vi "Dashboard Main.vi"() -> ()   [LabVIEW 2017]
uses:
  <vilib>/event_ctls.llb/eventvkey.ctl
  <vilib>/Rock Robotics/WPI/Dashboard/WPI_DashboardLogging Global.vi
  <vilib>/Utility/miscctls.llb/LVRowAndColumnTypeDef.ctl
  <vilib>/Rock Robotics/Network Tables/NT Read Boolean.vi
  <vilib>/Rock Robotics/Network Tables/NT Read Numeric Array.vi
panel:
  in  "Camera Settings Right":T1={"Frame Rate"=30, "Compression"=30, "Size"=1, "DB Camera Config"=FALSE} {"Frame Rate" scale=1.0..30.0; "Compression" scale=100.0..-1.0; "Size" items=["640x480", "320x240", "160x120"]}
  in  "Camera Name Right":string(combo)="No Camera Selection"
  out "Camera Info":cluster{"Mbps LED":bool, "Mbps":dbl, "fps":dbl} {"fps" format="%#.1g"; "Mbps" format="%#.1g"}
  in  "Camera Settings":T1={"Frame Rate"=30, "Compression"=30, "Size"=1, "DB Camera Config"=FALSE} {"Frame Rate" scale=1.0..30.0; "Compression" scale=100.0..-1.0; "Size" items=["640x480", "320x240", "160x120"]}
  in  "TCP":refnum<k5>
  in  "Rec Mode":enum32{"Stop", "Record", "Playback"}(radio)
  out "Robot IP":string
  out "Image Message":string="Timeout in Camera Communications"
  in  "Dashboard Tab":T2(tab)
  in  "Select Auto":string(combo)="Select Autonomous ..."
  out "NT Connection":bool
  out "MotorChart R":cluster{"Numeric":dbl, "Numeric":dbl}(graph)
  out "MotorChart L":cluster{"Numeric":dbl, "Numeric":dbl}(graph)
  out "MotorSliders R":cluster{"MotorSlide1":dbl, "MotorSlide2":dbl} {"MotorSlide2" scale=-1.0..1.0 scale format="%#_2e"; "MotorSlide1" scale=-1.0..1.0 scale format="%#_2e"}
  out "MotorSliders L":cluster{"MotorSlide1":dbl, "MotorSlide2":dbl} {"MotorSlide2" scale=-1.0..1.0 scale format="%#_2e"; "MotorSlide1" scale=-1.0..1.0 scale format="%#_2e"}
  out "JS1 Z":dbl(slide) scale=-1.0..1.0 scale format="%#_2e"
  out "JS1 Graph":cluster{"X":dbl, "Y":dbl}[](graph)
  out "JS1 Buttons":T3
  out "JS2 Z":dbl(slide) scale=-1.0..1.0 scale format="%#_2e"
  out "JS2 Graph":cluster{"X":dbl, "Y":dbl}[](graph)
  out "JS2 Buttons":T3
  out "Mode":T4(ring)=enum."Auto Disabled"
  out "Camera Image Right":T5(plugin-control)
  in  "DB/String 9":string
  in  "DB/String 8":string
  in  "DB/String 7":string
  in  "DB/String 6":string
  in  "DB/String 5":string
  in  "DB/String 4":string
  in  "DB/String 3":string
  in  "DB/String 2":string
  in  "DB/String 1":string
  in  "DB/String 0":string
  in  "DB/Slider 0":dbl(slide) scale=0.0..5.0
  in  "DB/Slider 1":dbl(slide) scale=0.0..5.0
  in  "DB/Slider 2":dbl(slide) scale=0.0..5.0
  in  "DB/Slider 3":dbl(slide) scale=0.0..5.0
  out "DB/LED 3":bool
  out "DB/LED 2":bool
  out "DB/LED 1":bool
  out "DB/LED 0":bool
  in  "DB/Button 3":bool
  in  "DB/Button 2":bool
  in  "DB/Button 1":bool
  in  "DB/Button 0":bool caption="New Name"
  in  "Test Slider":dbl(slide) scale=0.0..100.0 scale format="%#_3g"
  in  "On/Off":bool caption="Solenoid"
  in  "Test Name":u16(ring) items=["Select the test to run..."]
  in  "Test Tree":string(tree)
  in  "Motor":cluster{"Value":dbl, "Enable":bool} {"Value" scale=-1.0..1.0 scale format="%#_3g"}
  out "Progress":T6 {"Test Progress" scale=0.0..100.0}
  in  "Rev/Fwd":cluster{"Forward":bool, "Reverse":bool}
  in  "Test Ring":u16(ring) items=["Monochrome", "Color"]
  out "Cmd Status":string
  in  "Execute Command":bool
  in  "Command Params":string[][](table)
  in  "Command Selection":i32(listbox)
  in  "CheckList":i32(listbox)
  out "Tree":string(tree)
  out "Camera Image":T5(plugin-control)
  out "Background":bool
  in  "Camera Name":string(combo)="No Camera Selection"
  # "HW"
  # "HW"
  # "Drive Motors"
  # "Joysticks"
  # "Front"
  # "Right"
  # "Left"
  # "Back"
  # "This tab is a great place for autonomous settings and robot-specific values.\nPlace controls and indicators inside this tab and match name to\nDashboard Variables on robot. You can also delete this comment."
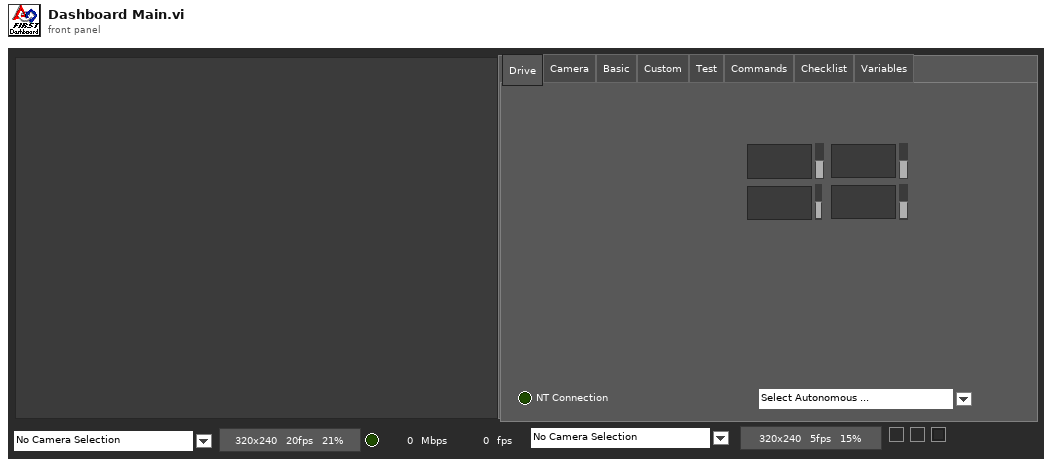
[diagram p1: front panel]
types:
  T1 = cluster{"Frame Rate":i32, "Compression":i32, "Size":u16, "DB Camera Config":bool}
  T2 = enum32{"Drive", "Camera", "Basic", "Custom", "Test", "Commands", "Checklist", "Variables"}
  T3 = cluster{bool, bool, bool, bool, bool, bool, bool, bool, bool, bool, bool, bool}
  T4 = enum8{"Tele-Op Disabled", "Tele-Op Enabled", "Auto Disabled", "Auto Enabled", "Test Disabled", "Test Enabled", "Disconnected", "No Code", "E-Stop"}
  T5 = typedef "IMAQ Image.ctl" = refnum<image>
  T6 = cluster{"Test Progress":u8, "Test Progress Text":string}
  T7 = cluster{"Save Path":path, "Interval (s)":dbl, "Keep":i32}
  T8 = typedef "Image Type" = u32
  T9 = cluster{"IDs":cluster{"RPC field ID":u16, "Unique ID":u16}, "String":string}
  T10 = cluster{"Error Strings":string, "Disable Counts":cluster{u16, u16}, "Rail Faults":cluster{u16, u16, u16}, "Robot IP":string, "DB Mode":u8, "Event Info":cluster{"Name":string, "Type":u8, "Number":u16, "Replay":u8}}
  T11 = cluster{"Storage":cluster{"Disk Free":u64, "RAM Block":u32, "RAM free":u32}, "CPU Utilization":cluster{"CPU % ISR":sgl, "CPU % Time Crit":sgl, "CPU % Timed Str":sgl, "CPU % High":sgl, "CPU % Above":sgl, "CPU % Normal":sgl, "CPU % Low":sgl}, "CAN":cluster{"% Bus Utilization":sgl, "Bus Off Cnt":u32, "TX_FIFO Full Cnt":u32, "Receive Error Cnt":u8, "Transmit Error Cnt":u8}, "HID":cluster{"HID Outputs":u32, "Rumble Low":u16, "Rumble High":u16}[]}
  T12 = cluster{"Status bits":cluster{"Test Mode":bool, "Autonomous":bool, "Enabled":bool, "Code Start":bool, "Brownout":bool, "Reserved 2":bool, "Reserved 3":bool, "E-Stop":bool}, "Code Trace":cluster{"Disabled":bool, "TeleOp":bool, "Auto":bool, "Test":bool}, "Controller Type":enum16{"unknown", "cRIO", "roboRio"}, "Code?":enum16{"unknown", "noCode", "code"}, "Battery V":dbl}
  T13 = cluster{"Control Bits":cluster{"TestMode":bool, "Autonomous":bool, "Enabled":bool, "FMS Present":bool, bool, bool, bool, "E-Stop":bool}, "Team Station ":u8, "Countdown":sgl, "Joystick Values":cluster{"Axes":dbl[], "Buttons":bool[], "POVs":i16[]}[]}
  T14 = cluster{"Axes":dbl[], "Buttons":bool[], "POVs":i16[]}[]
  T15 = cluster{"Axes":dbl[], "Buttons":bool[], "POVs":i16[]}
  T16 = cluster{"Buttons[0]":bool, "Buttons[1]":bool, "Buttons[2]":bool, "Buttons[3]":bool, "Buttons[4]":bool, "Buttons[5]":bool, "Buttons[6]":bool, "Buttons[7]":bool, "Buttons[8]":bool, "Buttons[9]":bool, "Buttons[10]":bool, "Buttons[11]":bool}
  T17 = cluster{"Camera Image":refnum<vi>, "Dashboard Tab":refnum<vi>, "Background":refnum<vi>, "Rec Mode":refnum<vi>, "Test Slider":refnum<vi>, "On/Off ":refnum<vi>, "Test Ring":refnum<vi>, "Rev/Fwd":refnum<vi>, "Test Name":refnum<vi>, "Motor":refnum<vi>, "Progress":refnum<vi>, "CheckList":refnum<vi>, "Tree":refnum<vi>, "Test Tree":refnum<vi>, "Command Params":refnum<vi>, "Command Selection":refnum<vi>, "Execute Command":refnum<vi>, "Cmd Status":refnum<vi>, "Camera Settings":refnum<vi>, "Camera Name":refnum<vi>, "Camera Info":refnum<vi>, "Camera Settings Right":refnum<vi>, "Camera Name Right":refnum<vi>, "Camera Image Right":refnum<vi>}
  T18 = cluster{"Camera Name":string, string, "Saved DB Images Info":cluster{"Save Path":path, "Interval (s)":dbl, "Keep":i32}}
  T19 = cluster{"Camera Name Right":string, string, "Saved DB Images Info":cluster{"Save Path":path, "Interval (s)":dbl, "Keep":i32}}
  T20 = cluster{"Operation":enum16{"Update", "Clear"}, "Color Box":u32}[]
  T21 = typedef "eventvkey.ctl" = enum16{"ASCII", "Enter", "Return", "Shift", "Ctrl", "Alt", "Cmd", "Opt", "Caps", "NumLock", "Clear", "Break", "Up", "Down", "Left", "Right", "Insert", "Delete", "Home", "End", "PageUp", "PageDown", "Escape", "Help", "Pause", "ScrollLock", "F1", "F2", "F3", "F4", "F5", "F6", "F7", "F8", "F9", "F10", "F11", "F12", "F13", "F14", "F15", "F16", "F17", "F18", "F19", "F20", "F21", "F22", "F23", "F24", "Play", "VolumeUp", "VolumeDown", "Mute", "Two Byte Char"}
  T22 = cluster{"Image Size":bool, "Image Type":bool, "Pixel Value":bool, "ROI Information":bool, "Zoom Factor":bool}
  T23 = cluster{"Operation":enum16{"Update", "Clear"}, "Color Box":u32}
  T24 = typedef "LVRowAndColumnTypeDef.ctl" = cluster{"Row":i32, "Column":i32}
  T25 = cluster{"Shift":bool, "Ctrl":bool, "Alt":bool, "Cmd":bool, "Opt":bool}
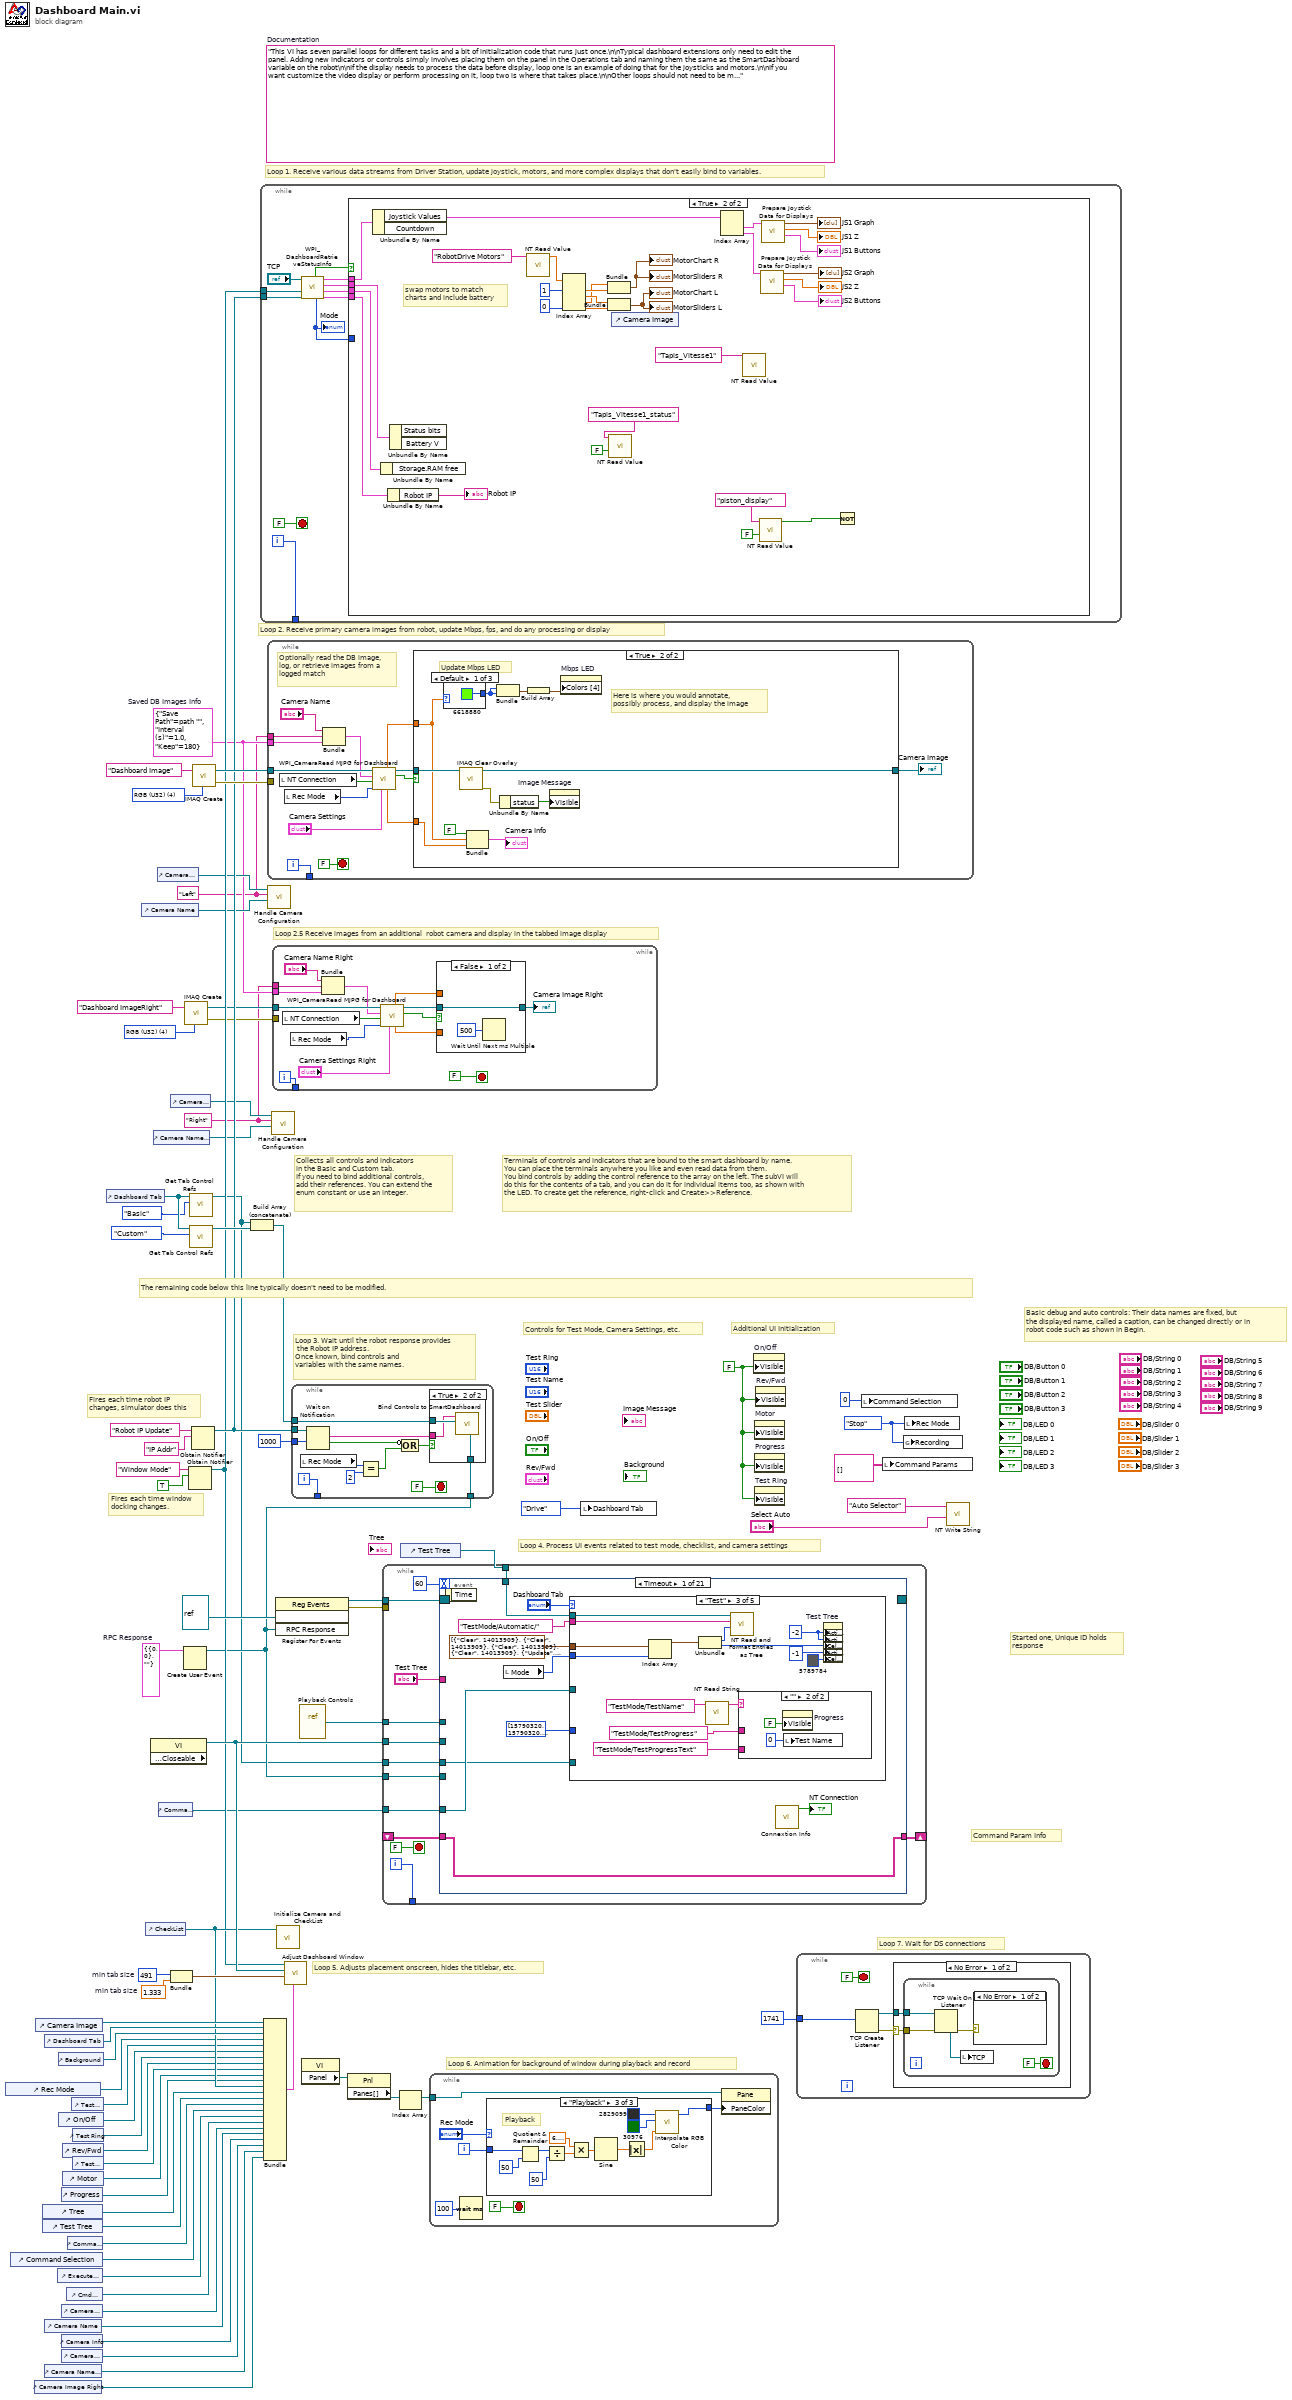
[diagram p0: block diagram]
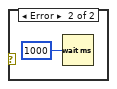
[diagram p3: hidden frame]
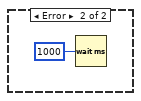
[diagram p4: hidden frame]
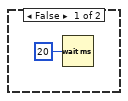
[diagram p5: hidden frame]
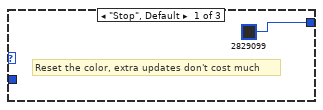
[diagram p6: hidden frame]
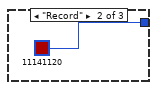
[diagram p7: hidden frame]
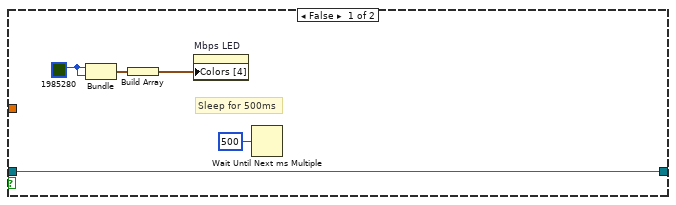
[diagram p9: hidden frame]
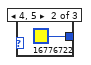
[diagram p10: hidden frame]
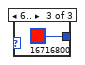
[diagram p11: hidden frame]
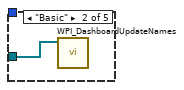
[diagram p13: hidden frame]
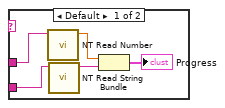
[diagram p14: hidden frame]
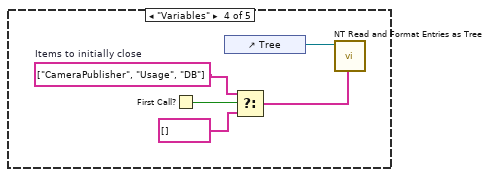
[diagram p15: hidden frame]
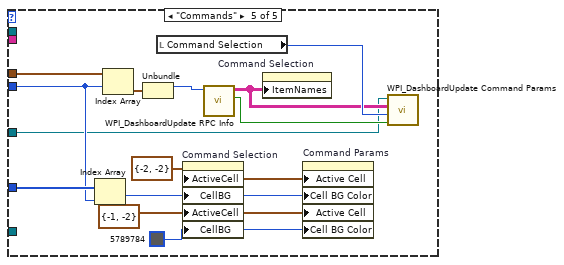
[diagram p16: hidden frame]
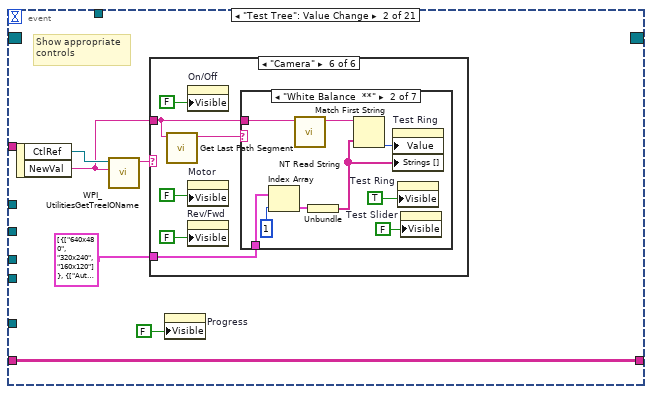
[diagram p17: hidden frame]
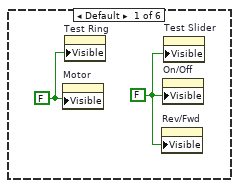
[diagram p18: hidden frame]
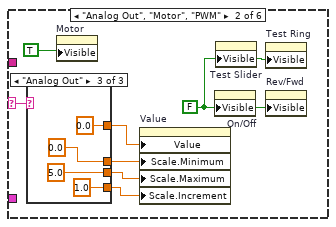
[diagram p19: hidden frame]
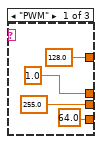
[diagram p20: hidden frame]
diagram:
  w3 = T7 {"Save Path"=path "", "Interval (s)"=1.0, "Keep"=180}  # Saved DB Images Info
  w2 = "Right"
  w1 = "Left"
  w13 = T8 4 items=["Grayscale (U8)", "Grayscale (I16)", "Grayscale (SGL)", "Complex (CSG)", "RGB (U32)", "HSL (U32)", "RGB (U64)"] ("Image Type")
  w29 = T9 {"IDs"={"RPC field ID"=0, "Unique ID"=0}, "String"=""}  # RPC Response
  w52 = 491  # min tab size
  w51 = 1.333  # min tab size
  w59 = enum32{"Stop", "Record", "Playback"}."Stop" ("Rec Mode")
  w36 = FALSE ("Visible")
  (unwired) "This VI has seven parallel loops for different tasks and a bit of initialization code that runs just once.\n\nTypical dashboard extensions only need to edit the panel. Adding new indicators or controls simply involves placing them on the panel in the Operations tab and naming them the same as the SmartDashboard variable on the robot\n\nIf the display needs to process the data before display, loop one is an example of doing that for the joysticks and motors.\n\nIf you want customize the video display or perform processing on it, loop two is where that takes place.\n\nOther loops should not need to be modified. They are pretty standard, and document the task they perform."  # Documentation
  w76 = T8 4 items=["Grayscale (U8)", "Grayscale (I16)", "Grayscale (SGL)", "Complex (CSG)", "RGB (U32)", "HSL (U32)", "RGB (U64)"] ("Image Type")
  # "Loop 2.5 Receive images from an additional  robot camera and display in the tabbed image display"
  # "Command Param Info"
  # "Started one, Unique ID holds\nresponse"
  # "Loop 7. Wait for DS connections"
  # "Basic debug and auto controls: Their data names are fixed, but\nthe displayed name, called a caption, can be changed directly or in\nrobot code such as shown in Begin."
  # "Controls for Test Mode, Camera Settings, etc."
  # "Additional UI Initialization"
  # "Loop 6. Animation for background of window during playback and record"
  # "Fires each time robot IP\nchanges, simulator does this"
  # "Fires each time window\ndocking changes."
  # "Collects all controls and indicators\nin the Basic and Custom tab.\nIf you need to bind additional controls,\nadd their references. You can extend the\nenum constant or use an integer."
  # "The remaining code below this line typically doesn't need to be modified."
  # "Loop 4. Process UI events related to test mode, checklist, and camera settings"
  # "Terminals of controls and indicators that are bound to the smart dashboard by name.\nYou can place the terminals anywhere you like and even read data from them.\nYou bind controls by adding the control reference to the array on the left. The subVI will\ndo this for the contents of a tab, and you can do it for individual items too, as shown with\nthe LED. To create get the reference, right-click and Create>>Reference."
  # "Loop 3. Wait until the robot response provides\n the Robot IP address.\nOnce known, bind controls and\nvariables with the same names."
  # "Loop 5. Adjusts placement onscreen, hides the titlebar, etc."
  # "Loop 1. Receive various data streams from Driver Station, update joystick, motors, and more complex displays that don't easily bind to variables."
  # "Loop 2. Receive primary camera images from robot, update Mbps, fps, and do any processing or display"
  n1 = control-ref of="Rec Mode"() -> (w42:refnum<vi>)
  n2 = control-ref of="Command Selection"() -> (w28:refnum<vi>)
  n3 = control-ref of="Camera Image Right"() -> (w6:refnum<vi>)
  n4 = control-ref of="Camera Image"() -> (w54:refnum<vi>)
  n5 = control-ref of="Tree"() -> (w46:refnum<vi>)
  n6 = control-ref of="Test Tree"() -> (w45:refnum<vi>)
  n7 = control-ref of="Dashboard Tab"() -> (w53:refnum<vi>)
  n8 = control-ref of="Camera Name"() -> (w19:refnum<vi>)
  n9 = control-ref of="Camera Name Right"() -> (w7:refnum<vi>)
  n10 = control-ref of="Execute Command"() -> (w30:refnum<vi>)
  n11 = control-ref of="Background"() -> (w49:refnum<vi>)
  n12 = control-ref of="On/Off"() -> (w40:refnum<vi>)
  n13 = control-ref of="Progress"() -> (w37:refnum<vi>)
  n14 = control-ref of="Camera Settings"() -> (w20:refnum<vi>)
  n15 = control-ref of="Camera Info"() -> (w18:refnum<vi>)
  n16 = control-ref of="Camera Settings Right"() -> (w8:refnum<vi>)
  n17 = control-ref of="Rev/Fwd"() -> (w38:refnum<vi>)
  n18 = control-ref of="Motor"() -> (w43:refnum<vi>)
  n19 = control-ref of="Cmd Status"() -> (w24:refnum<vi>)
  n20 = control-ref of="Command Params"() -> (w31:refnum<vi>)
  n21 = control-ref of="Test Slider"() -> (w41:refnum<vi>)
  n22 = control-ref of="Test Ring"() -> (w39:refnum<vi>)
  n23 = control-ref of="Test Name"() -> (w44:refnum<vi>)
  n24 = control-ref of="Dashboard Tab"() -> (w57:refnum<vi>)
  n25 = control-ref of="Camera Name"() -> (w21:refnum<vi>)
  n26 = control-ref of="CheckList"() -> (w47:refnum<vi>)
  n27 = property class="VI" props=["Front Panel.Closeable"]() -> (reference out=w58:refnum<vi>)  [unwired: 2 in, 2 out]
  n28 = control-ref of="Camera Name Right"() -> (w9:refnum<vi>)
  n29 = control-ref of="Camera Settings"() -> (w22:refnum<vi>)
  n30 = control-ref of="Command Params"() -> (w23:refnum<vi>)
  n31 = control-ref of="Camera Settings Right"() -> (w10:refnum<vi>)
  n32 = Bundle("min tab size"=w52, "min tab size"=w51) -> (w50:cluster{"min tab size":i32, "min tab size":dbl})  [unwired: 1 in]
  n33 = Create User Event(user event datatype=w29) -> (user event=w25:refnum<user-event>)  [unwired: 1 in, 1 out]
  n34 = call "IMAQ Create"("Image Name"="Dashboard ImageRight", "Image Type"=w13) -> ("New Image"=w12:T5, "error out"=w11:errorcluster)  [unwired: 2 in, 1 out]
  n35 = Obtain Notifier(name (unnamed)="Window Mode", notification data type=TRUE) -> (notifier out=w34:refnum<notifier>)  [unwired: 2 in, 2 out]
  n36 = call <vilib>:"Get Tab Control Refs.vi"("Page Index"=T2."Basic" ("Dashboard Tab"), "TabControl in"=w57) -> ("ControlsOnPage"=w17:refnum<vi>[])  [unwired: 9 in]
  n37 = call <vilib>:"Get Tab Control Refs.vi"("Page Index"=T2."Custom" ("Dashboard Tab"), "TabControl in"=w57) -> ("ControlsOnPage"=w56:refnum<vi>[])  [unwired: 9 in]
  n38 = Obtain Notifier(name (unnamed)="Robot IP Update", notification data type="IP Addr" ("name (unnamed)")) -> (notifier out=w35:refnum<notifier>)  [unwired: 2 in, 2 out]
  n39 = call "IMAQ Create"("Image Name"="Dashboard Image", "Image Type"=w76) -> ("New Image"=w74:T5, "error out"=w73:errorcluster)  [unwired: 2 in, 1 out]
  n40 = Build Array (concatenate)(w17, w56) -> (w55:refnum<vi>[])
  n41 = while {
    tunnel: [w86] -> _
    tunnel: w35 -> [w80]
    tunnel: w34 -> [w77]
    i -> [w86]
    stop <- FALSE stop-if-true
    n42 = call <vilib>:"WPI_DashboardRetrieveStatusInfo.vi"("Binding Refnum"=w80, "Window Mode Notifier"=w77, "TCP Cnx"="TCP") -> ("Power and Errors"=w81:T10, "Robot Metrics"=w84:T11, "Status Info"=w85:T12, "Control Info"=w82:T13, "Robot Mode"=w79:T4, "Process?"=w83:bool)  [unwired: 3 in]
    "Mode" <- w79
    n43 = case shown="True" w83 {
      tunnel: w85 -> [_ w120]
      tunnel: w84 -> [_ w119]
      tunnel: w82 -> [_ w118]
      tunnel: w81 -> [_ w117]
      tunnel: w79 -> [_ _]
      frame False {
        n44 = Wait (ms)(milliseconds to wait=u32 20) -> ()  [unwired: 1 out]
      }
      frame True {
        # "swap motors to match\ncharts and include battery"
        n45 = Unbundle By Name(w118) -> ("Joystick Values"=w108:T14)  [unwired: 1 out]
        n46 = Unbundle By Name(w119) -> ()  [unwired: 1 out]
        n47 = Unbundle By Name(w117) -> ("Robot IP"=→"Robot IP":string)
        n48 = Unbundle By Name(w120) -> ()  [unwired: 2 out]
        n49 = call-poly <vilib>:"NT Read Value.vi"("Name"="RobotDrive Motors") -> ("Numeric Array"=w98:dbl[])  [unwired: 9 in, 1 out]
        n50 = Index Array(array=w98, index #1=1, index #4=0) -> (element #1=w112:dbl, element #2=w113:dbl, element #3=w111:dbl, element #4=w116:dbl)  [unwired: 2 in]
        n51 = Bundle("Numeric"=w111, "Numeric"=w112) -> (→"MotorChart R" →"MotorSliders R":cluster{"Numeric":dbl, "Numeric":dbl})  [unwired: 1 in]
        n52 = Bundle("Numeric"=w113, "Numeric"=w116) -> (→"MotorChart L" →"MotorSliders L":cluster{"Numeric":dbl, "Numeric":dbl})  [unwired: 1 in]
        n53 = call-poly <vilib>:"NT Read Value.vi"("Default Value"=FALSE, "Name"="Tapis_Vitesse1_status") -> ()  [unwired: 8 in, 2 out]
        n54 = control-ref of="Camera Image"() -> ()  [unwired: 1 out]
        n55 = Index Array(array=w108) -> (element #1=w107:T15, element #2=w103:T15)  [unwired: 2 in]
        n56 = call-poly <vilib>:"NT Read Value.vi"("Name"="Tapis_Vitesse1") -> ("Numeric"=w90:dbl)  [unwired: 9 in, 1 out]
        n57 = call-poly <vilib>:"NT Read Value.vi"("Default Value"=FALSE, "Name"="piston_display") -> ("Boolean"=w96:bool)  [unwired: 8 in, 1 out]
        n58 = call "Prepare Joystick Data for Displays.vi"("Joystick Values"=w103) -> ("Buttons"=→"JS2 Buttons":T16, "Z Axis"=→"JS2 Z":dbl, "Cartesian Data"=→"JS2 Graph":cluster{"X axis":dbl, "X axis":dbl}[])  [unwired: 8 in]
        n59 = call "Prepare Joystick Data for Displays.vi"("Joystick Values"=w107) -> ("Buttons"=→"JS1 Buttons":T16, "Z Axis"=→"JS1 Z":dbl, "Cartesian Data"=→"JS1 Graph":cluster{"X axis":dbl, "X axis":dbl}[])  [unwired: 8 in]
        n60 = Not(x=w96) -> (.not. x?=w95:bool)
      }
    }
  }
  n61 = Bundle("Camera Image"=w54, "Dashboard Tab"=w53, "Background"=w49, "Rec Mode"=w42, "Test Slider"=w41, "On/Off"=w40, "Test Ring"=w39, "Rev/Fwd"=w38, "Test Name"=w44, "Motor"=w43, "Progress"=w37, "CheckList"=w47, "Tree"=w46, "Test Tree"=w45, "Command Params"=w31, "Command Selection"=w28, "Execute Command"=w30, "Cmd Status"=w24, "Camera Settings"=w20, "Camera Name"=w19, "Camera Info"=w18, "Camera Settings Right"=w8, "Camera Name Right"=w7, "Camera Image Right"=w6) -> (w48:T17)  [unwired: 1 in]
  n62 = call "Handle Camera Configuration.vi"("CameraNameRef"=w21, "Display Name"=w1, "ClusterRef"=w22) -> ()  [unwired: 9 in]
  n63 = while {
    tunnel: w74 -> [w133]
    tunnel: w73 -> [_]
    tunnel: [w134] -> _
    tunnel: w3 -> [w124]
    tunnel: w1 -> [w121]
    i -> [w134]
    stop <- FALSE stop-if-true
    # "Optionally read the DB image,\nlog, or retrieve images from a\nlogged match"
    n64 = local read "NT Connection"() -> (w125:bool)
    n65 = local read "Rec Mode"() -> (w129:enum32{"Stop", "Record", "Playback"})
    n66 = Bundle("Camera Name"="Camera Name", w121, "Saved DB Images Info"=w124) -> (w123:T18)  [unwired: 1 in]
    n67 = call <vilib>:"WPI_CameraRead MJPG for Dashboard.vi"("Camera Settings"="Camera Settings", "Rec Mode"=w129, "NT Connection"=w125, "Capture Info"=w123, "Refnum in"=w133) -> ("Active"=w131:bool, "Refnum out"=w132:T5, "FPS"=w130:dbl, "Bandwidth (Mbps)"=w128:dbl)  [unwired: 3 in]
    n68 = case shown="True" w131 {
      tunnel: w132 -> [w136 w147]
      tunnel: w128 -> [_ w144]
      tunnel: w130 -> [_ w145]
      tunnel: [w136 w141] -> w126
      frame False {
        w138 = u32 1985280 ("Color Box")
        # "Sleep for 500ms"
        n69 = Bundle("Color Box"=w138, "Color Box"=w138) -> (w139:cluster{"Color Box":u32, "Color Box":u32})  [unwired: 1 out]
        n70 = Build Array(w139) -> (w137:cluster{"Color Box":u32, "Color Box":u32}[])
        n71 = property on="Mbps LED" class="Bool (strict)"("Colors [4]"=w137) -> ()  [unwired: 2 in, 2 out]
        n72 = Wait Until Next ms Multiple(millisecond multiple=u32 500) -> ()  [unwired: 1 out]
      }
      frame True {
        # "Here is where you would annotate,\npossibly process, and display the image"
        # "Update Mbps LED"
        n73 = case shown="Default" w144 {
          tunnel: [u32 6618880 ("Color Box") u32 16776722 ("Color Box") u32 16716800 ("Color Box")] -> w148
          frame Default {
          }
          frame 4, 5 {
          }
          frame 6.. {
          }
        }
        n74 = call "IMAQ Clear Overlay"("Image"=w147) -> ("error out"=w150:errorcluster, "Image Out"=w141:T5)  [unwired: 2 in, 7 out]
        n75 = Bundle(FALSE, "Bandwidth (Mbps)"=w144, "FPS"=w145) -> (→"Camera Info":cluster{bool, "Bandwidth (Mbps)":dbl, "FPS":dbl})  [unwired: 1 in]
        n76 = Bundle("Color Box"=w148, "Color Box"=w148) -> (w149:cluster{"Color Box":u32, "Color Box":u32})  [unwired: 1 out]
        n77 = Unbundle By Name(w150) -> ("status"=w151:bool)
        n78 = Build Array(w149) -> (w146:cluster{"Color Box":u32, "Color Box":u32}[])
        n79 = property on="Image Message" class="Str"("Visible"=w151) -> ()  [unwired: 2 in, 2 out]
        n80 = property on="Mbps LED" class="Bool (strict)"("Colors [4]"=w146) -> ()  [unwired: 2 in, 2 out]
      }
    }
    "Camera Image" <- w126
  }
  n81 = call "Handle Camera Configuration.vi"("CameraNameRef"=w9, "Display Name"=w2, "ClusterRef"=w10) -> ()  [unwired: 9 in]
  n82 = while {
    tunnel: w12 -> [w169]
    tunnel: w11 -> [_]
    tunnel: [w164] -> _
    tunnel: w3 -> [w158]
    tunnel: w2 -> [w155]
    i -> [w164]
    stop <- FALSE stop-if-true
    n83 = local read "NT Connection"() -> (w159:bool)
    n84 = local read "Rec Mode"() -> (w168:enum32{"Stop", "Record", "Playback"})
    n85 = Bundle("Camera Name Right"="Camera Name Right", w155, "Saved DB Images Info"=w158) -> (w157:T19)  [unwired: 1 in]
    n86 = call <vilib>:"WPI_CameraRead MJPG for Dashboard.vi"("Camera Settings"="Camera Settings Right", "Rec Mode"=w168, "NT Connection"=w159, "Capture Info"=w157, "Refnum in"=w169) -> ("Active"=w163:bool, "Refnum out"=w166:T5, "FPS"=w161:dbl, "Bandwidth (Mbps)"=w162:dbl)  [unwired: 3 in]
    n87 = case shown="False" w163 {
      tunnel: w166 -> [w170 w172]
      tunnel: w162 -> [_ _]
      tunnel: w161 -> [_ _]
      tunnel: [w170 w172] -> w160
      frame False {
        n88 = Wait Until Next ms Multiple(millisecond multiple=u32 500) -> ()  [unwired: 1 out]
      }
      frame True {
      }
    }
    "Camera Image Right" <- w160
  }
  n89 = register-events(refnum<vi> refnum, w25) -> (reference out=w63:refnum<event-registration>, error out=w62:errorcluster)  [unwired: 2 in]
  n90 = call "Initialize Camera and CheckList.vi"("ListBox in"=w47) -> ()  [unwired: 11 in]
  n91 = call "Adjust Dashboard Window.vi"("Sizing Refnums"=w48, "Size Constraints"=w50, "VI"=w58, "WIn Mode"=w34) -> ()  [unwired: 8 in]
  n92 = while {
    tunnel: w55 -> [w184]
    tunnel: w35 -> [w182]
    tunnel: [w180] -> _
    tunnel: u32 1000 ("milliseconds to wait") -> [w179]
    tunnel: w25 -> [w173]
    i -> [w180]
    stop <- FALSE stop-if-true
    n93 = local read "Rec Mode"() -> (w175:enum32{"Stop", "Record", "Playback"})
    n94 = Wait on Notification(notifier=w182, timeout in ms (-1)=w179) -> (notification=w181:string, timed out?=w177:bool)  [unwired: 2 in, 2 out]
    n95 = Equal?(x=w175, y=u16 2 ("Rec Mode")) -> (x = y?=w176:bool)
    n96 = Compound Arithmetic op=OR(invert w177, w176) -> (w178:bool)
    n97 = case shown="True" w178 {
      tunnel: w184 -> [_ w187]
      tunnel: w181 -> [_ w186]
      tunnel: w173 -> [_ w185]
      frame False {
      }
      frame True {
        n98 = call <vilib>:"Bind Controls to SmartDashboard.vi"("RPC ref"=w185, "Bound Control Refs"=w187, "Server IP Address"=w186) -> ()  [unwired: 9 in]
      }
    }
  }
  n99 = vi-ref "Playback Controls.vi"() -> (w64:refnum<vi>)
  n100 = property class="VI"() -> ("Panel"=w66:refnum<vi>)  [unwired: 2 in, 2 out]
  n101 = property class="Pnl"(reference=w66) -> ("Panes[]"=w67:refnum<vi>[])  [unwired: 1 in, 2 out]
  n102 = Index Array(array=w67) -> (element=w65:refnum<vi>)  [unwired: 1 in]
  n103 = control-ref of="Test Tree"() -> (w68:refnum<vi>)
  n104 = while {
    tunnel: [w197] -> _
    tunnel: w68 -> [w196]
    tunnel: w64 -> [w195]
    tunnel: w63 -> [w194]
    tunnel: w62 -> [_]
    tunnel: w58 -> [w193]
    tunnel: w25 -> [w192]
    tunnel: w23 -> [w191]
    shift-right: [w190] -> _
    shift-left: _ -> [w189]
    tunnel: w17 -> [w188]
    i -> [w197]
    stop <- FALSE stop-if-true
    n105 = event shown="[0] Timeout" {
      selector: w194 -> [_ _ _ _ _ _ _ _ _ _ _ _ _ _ _ _ _ _ _ _ _]
      dyn-events: [_ _ _ _ _ _ _ _ _ _ _ _ _ _ _ _ w457 _ _ _ _] -> _
      timeout: u32 60 ("milliseconds to wait") -> [_ _ _ _ _ _ _ _ _ _ _ _ _ _ _ _ _ _ _ _ _]
      tunnel: w196 -> [w209 _ _ _ _ _ _ _ _ _ _ _ _ _ _ _ _ _ _ _ _]
      tunnel: "Test Tree" -> [_ _ _ _ _ _ _ _ _ _ _ w424 w432 w434 w438 w446 _ _ _ _ _]
      tunnel: w195 -> [_ _ _ _ _ _ _ _ _ _ _ _ _ _ _ _ w459 _ w477 _ _]
      tunnel: w193 -> [_ _ _ _ _ _ _ _ _ _ _ _ _ _ _ _ w455 _ _ _ _]
      tunnel: w192 -> [_ _ _ _ _ _ _ _ _ _ _ _ _ _ _ _ w453 _ _ _ _]
      tunnel: w191 -> [w204 _ _ _ _ _ w375 _ _ _ _ _ _ _ _ _ _ _ _ _ _]
      tunnel: [w203 w252 w354 w359 w368 w372 w373 w382 w392 w399 w411 w423 w430 w433 w437 w445 w452 w472 w474 w478 w491] -> w190
      tunnel: w189 -> [w203 w252 w354 w359 w368 w372 w373 _ _ w399 w411 w423 w430 w433 w437 w445 w452 w472 w474 w478 w491]
      tunnel: w188 -> [w201 _ _ _ _ _ _ _ _ _ _ _ _ _ _ _ _ _ _ _ _]
      event Timeout {
        n106 = event-data() -> ()  [unwired: 1 in, 1 out]
        n107 = local read "Mode"() -> (w206:T4)
        n108 = case shown="\"Test\"" "Dashboard Tab" {
          tunnel: w209 -> [_ _ w225 _ _]
          tunnel: "TestMode/Automatic/" ("Name Pattern") -> [_ _ w224 _ _]
          tunnel: T20 [{"Operation"=enum."Clear", "Color Box"=14013909}, {"Operation"=enum."Clear", "Color Box"=14013909}, {"Operation"=enum."Clear", "Color Box"=14013909}, {"Operation"=enum."Clear", "Color Box"=14013909}, {"Operation"=enum."Update", "Color Box"=14013909}, {"Operation"=enum."Update", "Color Box"=16777215}, {"Operation"=enum."Clear", "Color Box"=14013909}, {"Operation"=enum."Clear", "Color Box"=14013909}, {"Operation"=enum."Clear", "Color Box"=14013909}] -> [_ _ w217 _ w245]
          tunnel: w206 -> [_ _ w216 _ w244]
          tunnel: u32[] [15790320, 15790320, 15790320, 15790320, 16777215, 16777215, 15790320, 15790320, 15790320] -> [_ _ _ _ w250]
          tunnel: w204 -> [_ _ _ _ w238]
          tunnel: w201 -> [_ w211 _ _ _]
          frame "Custom", Default {
          }
          frame "Basic" {
            n109 = call <vilib>:"WPI_DashboardUpdateNames.vi"("Controls on Tab"=w211) -> ()  [unwired: 11 in]
          }
          frame "Test" {
            w223 = -2 ("Active Item:Row Number")
            n110 = Index Array(array=w217, index=w216) -> (element=w218:T23)
            n111 = Unbundle(w218) -> ("Operation"=w219:enum16{"Update", "Clear"}, "Color Box"=w220:u32)
            n112 = call <vilib>:"NT Read String.vi"("Name"="TestMode/TestName") -> ("String"=w214:string)  [unwired: 9 in, 1 out]
            n113 = call <vilib>:"NT Read and Format Entries as Tree.vi"("Operation"=w219, "Name Pattern"=w224, "Tree Refnum"=w225) -> ()  [unwired: 7 in, 2 out]
            n114 = case shown="\"\"" w214 {
              tunnel: "TestMode/TestProgress" ("Name") -> [w227 _]
              tunnel: "TestMode/TestProgressText" ("Name") -> [w226 _]
              frame Default {
                n115 = call <vilib>:"NT Read Number.vi"("Name"=w227) -> ("Numeric"=w228:dbl)  [unwired: 9 in, 1 out]
                n116 = call <vilib>:"NT Read String.vi"("Name"=w226) -> ("String"=w229:string)  [unwired: 9 in, 1 out]
                n117 = Bundle("Numeric"=w228, "String"=w229) -> (→"Progress":cluster{"Numeric":dbl, "String":string})  [unwired: 1 in]
              }
              frame "" {
                n118 = property on="Progress" class="Clust (strict)"("Visible"=FALSE) -> ()  [unwired: 2 in, 2 out]
                n119 = local write "Test Name"(u16 0) -> ()
              }
            }
            n120 = property on="Test Tree" class="Tree (strict)"("Active Item Row Number"=w223, "ActiveColNum"=w223, "CellBG"=w220, "Active Item Row Number"=-1 ("Active Item:Row Number"), "CellBG"=u32 5789784 ("Color Box")) -> ()  [unwired: 2 in, 2 out]
          }
          frame "Variables" {
            w235 = string[] ["CameraPublisher", "Usage", "DB"]  # Items to initially close
            n121 = First Call?() -> (First Call?: T/F=w236:bool)
            n122 = control-ref of="Tree"() -> (w237:refnum<vi>)
            n123 = Select(t=w235, s=w236, f=string[] []) -> (s? t:f=w233:string[])
            n124 = call <vilib>:"NT Read and Format Entries as Tree.vi"("Tags to  Close"=w233, "Tree Refnum"=w237) -> ()  [unwired: 8 in, 2 out]
          }
          frame "Commands" {
            w246 = u32 5789784 ("Color Box")
            w247 = T24 {"Row"=-1, "Column"=-2} ("Active Cell:Active Cell")
            w249 = T24 {"Row"=-2, "Column"=-2} ("Active Cell:Active Cell")
            n125 = Index Array(array=w250, index=w244) -> (element=w248:u32)
            n126 = Index Array(array=w245, index=w244) -> (element=w243:T23)
            n127 = Unbundle(w243) -> ("Operation"=w242:enum16{"Update", "Clear"})  [unwired: 1 out]
            n128 = local read "Command Selection"() -> (w241:i32)
            n129 = property on="Command Selection" class="MCListbox (strict)"("ActiveCell"=w249, "CellBG"=w248, "ActiveCell"=w247, "CellBG"=w246) -> ()  [unwired: 2 in, 2 out]
            n130 = call <vilib>:"WPI_DashboardUpdate RPC Info.vi"("Operation"=w242) -> ("update"=w240:bool, "commands"=w239:string[][])  [unwired: 9 in]
            n131 = property on="Command Selection" class="MCListbox (strict)"("ItemNames"=w239) -> ()  [unwired: 2 in, 2 out]
            n132 = property on="Command Params" class="Tbl (strict)"("Active Cell"=w249, "Cell BG Color"=w248, "Active Cell"=w247, "Cell BG Color"=w246) -> ()  [unwired: 2 in, 2 out]
            n133 = call <vilib>:"WPI_DashboardUpdate Command Params.vi"("Update"=w240, "NewVal"=w241, "Commands"=w239, "Param Tbl"=w238) -> ()  [unwired: 7 in, 1 out]
          }
        }
        n134 = call <vilib>:"Connextion Info.vi"() -> ("Connected"=→"NT Connection":bool)  [unwired: 10 in, 1 out]
      }
      event "Test Tree": Value Change {
        # "Show appropriate\ncontrols"
        n135 = event-data() -> ("CtlRef"=w255:refnum<vi>, "NewVal"=w253:string)  [unwired: 1 in]
        n136 = call <vilib>:"WPI_UtilitiesGetTreeIOName.vi"("NewVal"=w253, "TreeControl in"=w255) -> ("I/O Name"=w256:string)  [unwired: 9 in]
        n137 = case shown="\"Camera\"" w256 {
          selector: w256 -> [_ w263 _ w285 w294 _]
          tunnel: w253 -> [_ _ w282 w284 _ w301]
          tunnel: cluster{string[]}[] [{["640x480", "320x240", "160x120"]}, {["Auto", "Fixed indoor", "Fixed outdoor 1", "Fixed outdoor 2", "Fixed fluorescent 1", "Fixed fluorescent 2", "Hold current"]}, {["Auto", "Flicker-free 50 Hz", "Flicker-free 60 Hz", "Hold current"]}, {["None", "Prioritize frame rate", "Prioritize image quality"]}, {["Monochrome", "Color"]}] -> [_ _ _ _ _ w300]
          frame Default {
            w258 = FALSE ("Visible")
            w257 = FALSE ("Visible")
            n138 = property on="Motor" class="Clust (strict)"("Visible"=w257) -> ()  [unwired: 2 in, 2 out]
            n139 = property on="Test Ring" class="Ring (strict)"("Visible"=w257) -> ()  [unwired: 2 in, 2 out]
            n140 = property on="Rev/Fwd" class="Clust (strict)"("Visible"=w258) -> ()  [unwired: 2 in, 2 out]
            n141 = property on="On/Off" class="Bool (strict)"("Visible"=w258) -> ()  [unwired: 2 in, 2 out]
            n142 = property on="Test Slider" class="Slide (strict)"("Visible"=w258) -> ()  [unwired: 2 in, 2 out]
          }
          frame "Analog Out", "Motor", "PWM" {
            w264 = FALSE ("Visible")
            n143 = case shown="\"Analog Out\"" w263 {
              tunnel: [1.0 ("Value") -1.0 ("Value") 0.0 ("Value")] -> w262
              tunnel: [255.0 ("Value") 1.0 ("Value") 5.0 ("Value")] -> w261
              tunnel: [128.0 ("Value") 0.0 ("Value") 0.0 ("Value")] -> w260
              tunnel: [64.0 ("Value") 0.5 ("Value") 1.0 ("Value")] -> w259
              frame "PWM" {
              }
              frame "Motor", Default {
              }
              frame "Analog Out" {
              }
            }
            n144 = property on="Motor" class="Clust (strict)"("Visible"=TRUE) -> ()  [unwired: 2 in, 2 out]
            n145 = property on="Value" class="Slide (strict)"("Value"=w260, "Scale.Minimum"=w262, "Scale.Maximum"=w261, "Scale.Increment"=w259) -> ()  [unwired: 2 in, 2 out]
            n146 = property on="On/Off" class="Bool (strict)"("Visible"=w264) -> ()  [unwired: 2 in, 2 out]
            n147 = property on="Test Slider" class="Slide (strict)"("Visible"=w264) -> ()  [unwired: 2 in, 2 out]
            n148 = property on="Test Ring" class="Ring (strict)"("Visible"=w264) -> ()  [unwired: 2 in, 2 out]
            n149 = property on="Rev/Fwd" class="Clust (strict)"("Visible"=w264) -> ()  [unwired: 2 in, 2 out]
          }
          frame "Servo" {
            w280 = FALSE ("Visible")
            n150 = call <vilib>:"NT Read Number.vi"("Name"=w282) -> ("Numeric"=w281:dbl)  [unwired: 9 in, 1 out]
            n151 = property on="Test Slider" class="Slide (strict)"("Visible"=TRUE, "Scale.Maximum"=170.0 ("Scale.Range:Maximum")) -> ()  [unwired: 2 in, 2 out]
            n152 = local write "Test Slider"(w281) -> ()
            n153 = property on="Motor" class="Clust (strict)"("Visible"=w280) -> ()  [unwired: 2 in, 2 out]
            n154 = property on="Rev/Fwd" class="Clust (strict)"("Visible"=w280) -> ()  [unwired: 2 in, 2 out]
            n155 = property on="On/Off" class="Bool (strict)"("Visible"=w280) -> ()  [unwired: 2 in, 2 out]
            n156 = property on="Test Ring" class="Ring (strict)"("Visible"=w280) -> ()  [unwired: 2 in, 2 out]
          }
          frame "Relay", "Solenoid" {
            w283 = FALSE ("Visible")
            n157 = property on="Motor" class="Clust (strict)"("Visible"=w283) -> ()  [unwired: 2 in, 2 out]
            n158 = property on="Test Slider" class="Slide (strict)"("Visible"=w283) -> ()  [unwired: 2 in, 2 out]
            n159 = Search and Replace String(input string=w284, search string="/Value  **", replace string="/Direction") -> (result string=w290:string)  [unwired: 5 in, 3 out]
            n160 = property on="Test Ring" class="Ring (strict)"("Visible"=w283) -> ()  [unwired: 2 in, 2 out]
            n161 = call <vilib>:"NT Read String.vi"("Name"=w290) -> ("String"=w288:string)  [unwired: 9 in, 1 out]
            n162 = Equal?(x="Both directions", y=w288) -> (x = y?=w286:bool)
            n163 = Not(x=w286) -> (.not. x?=w287:bool)
            n164 = property on="Rev/Fwd" class="Clust (strict)"("Visible"=w286) -> ()  [unwired: 2 in, 2 out]
            n165 = property on="On/Off" class="Bool (strict)"("Visible"=w287, "Caption.Text"=w285) -> ()  [unwired: 2 in, 2 out]
          }
          frame "Compressor", "Digital Out" {
            w293 = FALSE ("Visible")
            # "Get direction and finish"
            n166 = property on="Motor" class="Clust (strict)"("Visible"=w293) -> ()  [unwired: 2 in, 2 out]
            n167 = property on="Test Slider" class="Slide (strict)"("Visible"=w293) -> ()  [unwired: 2 in, 2 out]
            n168 = property on="Test Ring" class="Ring (strict)"("Visible"=w293) -> ()  [unwired: 2 in, 2 out]
            n169 = property on="On/Off" class="Bool (strict)"("Visible"=TRUE, "Caption.Text"=w294) -> ()  [unwired: 2 in, 2 out]
            n170 = property on="Rev/Fwd" class="Clust (strict)"("Visible"=FALSE) -> ()  [unwired: 2 in, 2 out]
          }
          frame "Camera" {
            n171 = call <vilib>:"Get Last Path Segment.vi"("String in"=w301) -> ("String out"=w302:string)  [unwired: 10 in]
            n172 = property on="On/Off" class="Bool (strict)"("Visible"=FALSE) -> ()  [unwired: 2 in, 2 out]
            n173 = property on="Motor" class="Clust (strict)"("Visible"=FALSE) -> ()  [unwired: 2 in, 2 out]
            n174 = property on="Rev/Fwd" class="Clust (strict)"("Visible"=FALSE) -> ()  [unwired: 2 in, 2 out]
            n175 = case shown="\"White Balance  **\"" w302 {
              tunnel: w301 -> [w308 w317 w326 w335 w344 _ w350]
              tunnel: w300 -> [w306 w314 w323 w332 w341 _ _]
              frame "Size  **" {
                n176 = Index Array(array=w306) -> (element=w305:cluster{string[]})  [unwired: 1 in]
                n177 = call <vilib>:"NT Read String.vi"("Name"=w308) -> ("String"=w307:string)  [unwired: 9 in, 1 out]
                n178 = Unbundle(w305) -> (w303:string[])
                n179 = Match First String(2:w303, 3:w307) -> (0:w304:i32)  [unwired: 1 out]
                n180 = property on="Test Ring" class="Ring (strict)"("Value"=w304, "Strings []"=w303) -> ()  [unwired: 2 in, 2 out]
                n181 = property on="Test Ring" class="Ring (strict)"("Visible"=TRUE) -> ()  [unwired: 2 in, 2 out]
                n182 = property on="Test Slider" class="Slide (strict)"("Visible"=FALSE) -> ()  [unwired: 2 in, 2 out]
              }
              frame "White Balance  **" {
                n183 = Index Array(array=w314, index=1) -> (element=w315:cluster{string[]})
                n184 = call <vilib>:"NT Read String.vi"("Name"=w317) -> ("String"=w316:string)  [unwired: 9 in, 1 out]
                n185 = Unbundle(w315) -> (w312:string[])
                n186 = Match First String(2:w312, 3:w316) -> (0:w311:i32)  [unwired: 1 out]
                n187 = property on="Test Ring" class="Ring (strict)"("Value"=w311, "Strings []"=w312) -> ()  [unwired: 2 in, 2 out]
                n188 = property on="Test Ring" class="Ring (strict)"("Visible"=TRUE) -> ()  [unwired: 2 in, 2 out]
                n189 = property on="Test Slider" class="Slide (strict)"("Visible"=FALSE) -> ()  [unwired: 2 in, 2 out]
              }
              frame "Exposure  **" {
                n190 = Index Array(array=w323, index=2) -> (element=w324:cluster{string[]})
                n191 = call <vilib>:"NT Read String.vi"("Name"=w326) -> ("String"=w325:string)  [unwired: 9 in, 1 out]
                n192 = Unbundle(w324) -> (w320:string[])
                n193 = Match First String(2:w320, 3:w325) -> (0:w321:i32)  [unwired: 1 out]
                n194 = property on="Test Ring" class="Ring (strict)"("Value"=w321, "Strings []"=w320) -> ()  [unwired: 2 in, 2 out]
                n195 = property on="Test Ring" class="Ring (strict)"("Visible"=TRUE) -> ()  [unwired: 2 in, 2 out]
                n196 = property on="Test Slider" class="Slide (strict)"("Visible"=FALSE) -> ()  [unwired: 2 in, 2 out]
              }
              frame "Exposure Priority  **" {
                n197 = Index Array(array=w332, index=3) -> (element=w333:cluster{string[]})
                n198 = call <vilib>:"NT Read String.vi"("Name"=w335) -> ("String"=w334:string)  [unwired: 9 in, 1 out]
                n199 = Unbundle(w333) -> (w329:string[])
                n200 = Match First String(2:w329, 3:w334) -> (0:w330:i32)  [unwired: 1 out]
                n201 = property on="Test Ring" class="Ring (strict)"("Value"=w330, "Strings []"=w329) -> ()  [unwired: 2 in, 2 out]
                n202 = property on="Test Ring" class="Ring (strict)"("Visible"=TRUE) -> ()  [unwired: 2 in, 2 out]
                n203 = property on="Test Slider" class="Slide (strict)"("Visible"=FALSE) -> ()  [unwired: 2 in, 2 out]
              }
              frame "Color Enable  **" {
                n204 = Index Array(array=w341, index=4) -> (element=w342:cluster{string[]})
                n205 = call <vilib>:"NT Read String.vi"("Name"=w344) -> ("String"=w343:string)  [unwired: 9 in, 1 out]
                n206 = Unbundle(w342) -> (w338:string[])
                n207 = Match First String(2:w338, 3:w343) -> (0:w339:i32)  [unwired: 1 out]
                n208 = property on="Test Ring" class="Ring (strict)"("Value"=w339, "Strings []"=w338) -> ()  [unwired: 2 in, 2 out]
                n209 = property on="Test Ring" class="Ring (strict)"("Visible"=TRUE) -> ()  [unwired: 2 in, 2 out]
                n210 = property on="Test Slider" class="Slide (strict)"("Visible"=FALSE) -> ()  [unwired: 2 in, 2 out]
              }
              frame Default {
                n211 = property on="Test Ring" class="Ring (strict)"("Visible"=FALSE) -> ()  [unwired: 2 in, 2 out]
                n212 = property on="Test Slider" class="Slide (strict)"("Visible"=FALSE) -> ()  [unwired: 2 in, 2 out]
              }
              frame "Brightness  **", "Color Level  **", "Compression  **", "FPS  **", "Sharpness  **" {
                n213 = call <vilib>:"NT Read Number.vi"("Name"=w350) -> ("Numeric"=w349:dbl)  [unwired: 9 in, 1 out]
                n214 = local write "Test Slider"(w349) -> ()
                n215 = property on="Test Slider" class="Slide (strict)"("Visible"=TRUE, "Scale.Maximum"=100.0 ("Scale.Range:Maximum")) -> ()  [unwired: 2 in, 2 out]
                n216 = property on="Test Ring" class="Ring (strict)"("Visible"=FALSE) -> ()  [unwired: 2 in, 2 out]
              }
            }
          }
        }
        n217 = property on="Progress" class="Clust (strict)"("Visible"=FALSE) -> ()  [unwired: 2 in, 2 out]
      }
      event "Test Name": Mouse Enter {
        # "Populate the ring with the list of tests"
        n218 = event-data() -> ()  [unwired: 1 in, 1 out]
        n219 = call <vilib>:"NT Read String Array.vi"("Name"="TestMode/TestList") -> ("String Array"=w358:string[])  [unwired: 9 in, 1 out]
        n220 = Build Array (concatenate)("Select the test to run...", w358) -> (w357:string[])
        n221 = property on="Test Name" class="Ring (strict)"("Strings []"=w357) -> ()  [unwired: 2 in, 2 out]
      }
      event "Test Name": Value Change {
        w360 = FALSE ("Visible")
        # "Tell the robot the test name to run"
        n222 = event-data() -> ("NewVal"=w364:u16)  [unwired: 1 in]
        n223 = property on="Test Name" class="Ring (strict)"() -> ("Strings []"=w365:string[])  [unwired: 2 in, 2 out]
        n224 = local write "Progress"(T6 {"Test Progress"=0, "Test Progress Text"=""} ("Progress")) -> ()
        n225 = Index Array(array=w365, index=w364) -> (element=w363:string)
        n226 = call <vilib>:"NT Write String.vi"("String"=w363, "Name"="TestMode/TestName") -> ()  [unwired: 9 in, 1 out]
        n227 = property on="Progress" class="Clust (strict)"("Visible"=TRUE) -> ()  [unwired: 2 in, 2 out]
        n228 = property on="Motor" class="Clust (strict)"("Visible"=w360) -> ()  [unwired: 2 in, 2 out]
        n229 = property on="Test Slider" class="Slide (strict)"("Visible"=w360) -> ()  [unwired: 2 in, 2 out]
        n230 = property on="On/Off" class="Bool (strict)"("Visible"=w360) -> ()  [unwired: 2 in, 2 out]
        n231 = property on="Rev/Fwd" class="Clust (strict)"("Visible"=w360) -> ()  [unwired: 2 in, 2 out]
        n232 = property on="Test Ring" class="Ring (strict)"("Visible"=w360) -> ()  [unwired: 2 in, 2 out]
      }
      event "Select Auto": Mouse Enter {
        # "Populate the combo box with the list of autonomous options"
        n233 = event-data() -> ()  [unwired: 1 in, 1 out]
        n234 = call <vilib>:"NT Read String Array.vi"("Name"="Auto List") -> ("String Array"=w367:string[])  [unwired: 9 in, 1 out]
        n235 = property on="Select Auto" class="CmbBox"("Strings[]"=w367) -> ()  [unwired: 2 in, 2 out]
      }
      event "Select Auto": Value Change {
        # "User modified the Auto Selection. Write to NT variable so robot knows."
        n236 = event-data() -> ("NewVal"=w370:string)  [unwired: 1 in]
        n237 = call <vilib>:"NT Write String.vi"("String"=w370, "Name"="Auto Selector") -> ()  [unwired: 9 in, 1 out]
      }
      event "Command Selection": Value Change {
        # "Get the params and show in table"
        n238 = event-data() -> ("NewVal"=w376:i32)  [unwired: 1 in]
        n239 = property on="Command Selection" class="MCListbox (strict)"() -> ("ItemNames"=w374:string[][])  [unwired: 2 in, 2 out]
        n240 = call <vilib>:"WPI_DashboardUpdate Command Params.vi"("NewVal"=w376, "Commands"=w374, "Param Tbl"=w375) -> ()  [unwired: 8 in, 1 out]
      }
      event "Execute Command": Value Change {
        # "Started one, Unique ID holds\nresponse"
        n241 = event-data() -> ()  [unwired: 1 in, 1 out]
        n242 = property on="Command Selection" class="MCListbox (strict)"() -> ("ItemNames"=w387:string[][])  [unwired: 2 in, 2 out]
        n243 = Index Array(array=w387, index (row)="Command Selection", index (col)=0) -> (element=w385:string)
        n244 = call <vilib>:"Invoke Commands.vi"("Command Params"="Command Params", "Function Name"=w385) -> ("Params"=w381:u8, "Started"=w380:bool)  [unwired: 7 in, 1 out]
        n245 = Array Subset(array="Command Params", length (row)=w381) -> (w382:string[][])  [unwired: 3 in]
        n246 = Select(t="Executing" ("Cmd Status"), s=w380, f="" ("Cmd Status")) -> (s? t:f=→"Cmd Status":string)
      }
      event "Command Selection": Double Click {
        n247 = event-data() -> ("Row"=w395:i32)  [unwired: 1 in]
        n248 = property on="Command Selection" class="MCListbox (strict)"() -> ("ItemNames"=w398:string[][])  [unwired: 2 in, 2 out]
        n249 = local read "Command Params"() -> (w394:string[][])
        n250 = Index Array(array=w398, index (row)=w395, index (col)=0) -> (element=w396:string)
        n251 = call <vilib>:"Invoke Commands.vi"("Command Params"=w394, "Function Name"=w396) -> ("Params"=w393:u8, "Started"=w388:bool)  [unwired: 7 in, 1 out]
        n252 = Array Subset(array=w394, length (row)=w393) -> (w392:string[][])  [unwired: 3 in]
        n253 = Select(t="Executing" ("Cmd Status"), s=w388, f="" ("Cmd Status")) -> (s? t:f=w389:string)
        n254 = local write "Cmd Status"(w389) -> ()
      }
      event "CheckList": Double Click {
        # "Shift clears all"
        # "Update symbols on the listbox"
        n255 = event-data() -> ("PlatMods.Shift"=w400:bool, "Row"=w402:i32)  [unwired: 1 in]
        n256 = case shown="True" w400 {
          tunnel: w402 -> [w406 _]
          tunnel: 1 -> [w405 _]
          frame False {
            n257 = property on="CheckList" class="LstBox (strict)"() -> ("Item Symbols"=w404:i32[])  [unwired: 2 in, 2 out]
            n258 = Replace Array Subset(array=w404, new element=w405, index=w406) -> (w403:i32[])
            n259 = property on="CheckList" class="LstBox (strict)"("Item Symbols"=w403) -> ()  [unwired: 2 in, 2 out]
          }
          frame True {
            w407 = 0 ("Top Row")
            n260 = property on="CheckList" class="LstBox (strict)"() -> ("Number of Rows"=w409:u32)  [unwired: 2 in, 2 out]
            n261 = Initialize Array(0, w409) -> (w408:i32[])
            n262 = property on="CheckList" class="LstBox (strict)"("Top Row"=w407, "Value"=w407, "Item Symbols"=w408) -> ()  [unwired: 2 in, 2 out]
          }
        }
      }
      event "CheckList": Key Down {
        # "Update symbols on the listbox\nLeft and right keys check and uncheck"
        n263 = event-data() -> ("VKey"=w413:T21)  [unwired: 1 in]
        n264 = case shown="\"Left\", \"Right\"" w413 {
          selector: w413 -> [w418 _]
          tunnel: eventvkey."Left" ("VKey") -> [w416 _]
          frame "Left", "Right" {
            n265 = Equal?(x=w416, y=w418) -> (x = y?=w417:bool)
            n266 = Select(t=0, s=w417, f=1) -> (s? t:f=w419:i32)
            n267 = property on="CheckList" class="LstBox (strict)"() -> ("Item Symbols"=w422:i32[])  [unwired: 2 in, 2 out]
            n268 = Replace Array Subset(array=w422, new element=w419, index="CheckList") -> (w421:i32[])
            n269 = property on="CheckList" class="LstBox (strict)"("Item Symbols"=w421) -> ()  [unwired: 2 in, 2 out]
          }
          frame Default {
          }
        }
      }
      event "Motor.Enable": Value Change {
        # "When the test mode otor enable helper is set, update that\ntree row item's value"
        n270 = event-data() -> ("NewVal"=w428:bool)  [unwired: 1 in]
        n271 = Unbundle("Motor") -> ("Value"=w427:dbl)  [unwired: 1 out]
        n272 = Select(t=w427, s=w428, f=0.0) -> (s? t:f=w425:dbl)
        n273 = call <vilib>:"NT Write Number.vi"("Numeric"=w425, "Name"=w424) -> ()  [unwired: 9 in, 1 out]
      }
      event "Test Slider": Value Change {
        # "When the test mode slider helper is set, update that\ntree row item's value"
        n274 = event-data() -> ("NewVal"=w431:dbl)  [unwired: 1 in]
        n275 = call <vilib>:"NT Write Number.vi"("Numeric"=w431, "Name"=w432) -> ()  [unwired: 9 in, 1 out]
      }
      event "On/Off": Value Change {
        # "When the test mode on/off helper value is set, update that\ntree row item's value"
        n276 = event-data() -> ("NewVal"=w436:bool)  [unwired: 1 in]
        n277 = Boolean To (0,1)(Boolean=w436) -> (0, 1=w435:i16)
        n278 = call <vilib>:"NT Write Number.vi"("Numeric"=w435, "Name"=w434) -> ()  [unwired: 9 in, 1 out]
      }
      event "Rev/Fwd": Value Change {
        # "When the test mode helper value for relays is set, update that\ntree row item's value"
        n279 = event-data() -> ("NewVal.Forward"=w444:bool, "NewVal.Reverse"=w443:bool)  [unwired: 1 in]
        n280 = Boolean To (0,1)(Boolean=w444) -> (0, 1=w440:i16)
        n281 = Boolean To (0,1)(Boolean=w443) -> (0, 1=w442:i16)
        n282 = Negate(x=w442) -> (-x=w441:i16)
        n283 = Add(x=w440, y=w441) -> (x+y=w439:i16)
        n284 = call <vilib>:"NT Write Number.vi"("Numeric"=w439, "Name"=w438) -> ()  [unwired: 9 in, 1 out]
      }
      event "Test Ring": Value Change {
        # "When a test mode helper value is selected from the ring,\nset the tree item's variable to the string value"
        n285 = event-data() -> ("NewVal"=w448:u16)  [unwired: 1 in]
        n286 = property on="Test Ring" class="Ring (strict)"() -> ("Strings []"=w449:string[])  [unwired: 2 in, 2 out]
        n287 = Index Array(array=w449, index=w448) -> (element=w447:string)
        n288 = call <vilib>:"NT Write String.vi"("String"=w447, "Name"=w446) -> ()  [unwired: 9 in, 1 out]
      }
      event "Rec Mode": Value Change {
        # "Update globals for recording mode and path to read log from.\nClear when logging and let NetworkTables set path for vision to\nuse."
        n289 = event-data() -> ("NewVal"=w460:enum32{"Stop", "Record", "Playback"})  [unwired: 1 in]
        n290 = global write "WPI_DashboardLogging Global.vi" "Logging Filename"(path "") -> ()
        n291 = global write "WPI_DashboardLogging Global.vi" "Recording"(w460) -> ()
        n292 = case shown="\"Playback\"" w460 {
          tunnel: w459 -> [_ w462 w471]
          tunnel: [_ _ w470] -> w457
          tunnel: [_ _ w469] -> _
          tunnel: w455 -> [_ _ w467]
          tunnel: cluster{i32, i32} {-250, 170} -> [_ _ w466]
          tunnel: [_ _ T22 {"Image Size"=TRUE, "Image Type"=TRUE, "Pixel Value"=TRUE, "ROI Information"=TRUE, "Zoom Factor"=FALSE} ("Image Information Shown:All Elements")] -> w450
          tunnel: [_ _ TRUE ("Zoom Factor")] -> w451
          tunnel: w453 -> [_ _ w463]
          frame Default {
          }
          frame "Stop", "Record" {
            # "Place Window too"
            n293 = invoke class="VI" method="FP.Close"(reference=w462) -> (reference out=w461:refnum<vi>)  [unwired: 2 in, 2 out]
            n294 = invoke class="VI" method="Abort VI"(reference=w461) -> ()  [unwired: 2 in, 3 out]
          }
          frame "Playback" {
            n295 = call "Open Playback Panel.vi"("Offset"=w466, "DB VI Ref"=w467, "Playback in"=w471) -> ("Playback out"=w468:refnum<vi>)  [unwired: 8 in]
            n296 = register-events(w468, w463) -> (reference out=w470:refnum<event-registration>, error out=w469:errorcluster)  [unwired: 2 in]
          }
        }
        n297 = property on="Camera Image Right" class="ImageControl"("Image Information Shown"=w450, "Image Information Visible"=w451) -> ()  [unwired: 2 in, 2 out]
        n298 = property on="Camera Image" class="ImageControl"("Image Information Shown"=w450, "Image Information Visible"=w451) -> ()  [unwired: 2 in, 2 out]
        n299 = call <vilib>:"WPI_DashboardNT Log FieldName Cache.vi"("Operation"=enum16{"Lookup/Add", "Index", "Clear"}."Clear") -> ()  [unwired: 8 in, 3 out]
      }
      event Panel Close {
        w473 = enum32{"Stop", "Record", "Playback"}."Stop" ("Rec Mode")
        # "Playback window has been closed, abort"
        n300 = event-data() -> ()  [unwired: 1 in, 4 out]
        n301 = local write "Rec Mode"(w473) -> ()
        n302 = global write "WPI_DashboardLogging Global.vi" "Recording"(w473) -> ()
      }
      event Panel Close {
        # "Abort playback window and ourself"
        n303 = event-data() -> ()  [unwired: 1 in, 4 out]
        n304 = invoke class="VI" method="FP.Close"(reference=w477) -> (reference out=w476:refnum<vi>)  [unwired: 2 in, 2 out]
        n305 = invoke class="VI" method="Abort VI"(reference=w476) -> (error out=w475:errorcluster)  [unwired: 2 in, 2 out]
        n306 = invoke class="VI" method="Abort VI"(error in=w475) -> ()  [unwired: 2 in, 3 out]
      }
      event User Event {
        n307 = event-data() -> ("IDs"=w484:cluster{"RPC field ID":u16, "Unique ID":u16}, "String"=w483:string)  [unwired: 1 in]
        n308 = Bundle("IDs"=w484, "String"=w483) -> (w482:T9)  [unwired: 1 in]
        n309 = call <vilib>:"Retrieve RPC Response.vi"("RPC Response"=w482) -> ("Output"=w480:string[][])  [unwired: 10 in]
        n310 = Build Array (concatenate)(w478, w480) -> (w479:string[][])
        n311 = local write "Command Params"(w479) -> ()
        n312 = local write "Cmd Status"("" ("Cmd Status")) -> ()
      }
      event "Tree": Double Click {
        n313 = event-data() -> ("PlatMods"=w490:T25, "Tag"=w487:string)  [unwired: 1 in]
        n314 = Unbundle(w490) -> ("Shift"=w489:bool)  [unwired: 4 out]
        n315 = String Subset(string=w487, length (rest)=1 ("length (rest)")) -> (substring=w486:string)  [unwired: 1 in]
        n316 = Not(x=w489) -> (.not. x?=w488:bool)
        n317 = case shown="\"/\"" w486 {
          tunnel: w487 -> [_ w493]
          tunnel: w488 -> [_ w492]
          frame Default {
          }
          frame "/" {
            n318 = call <vilib>:"NT Update Persistence.vi"("Persistence"=w492, "Name"=w493) -> ()  [unwired: 9 in, 1 out]
          }
        }
      }
    }
  }
  n319 = while {
    tunnel: w65 -> [w495]
    i -> [w498]
    stop <- FALSE stop-if-true
    n320 = Wait (ms)(milliseconds to wait=u32 100) -> ()  [unwired: 1 out]
    n321 = case shown="\"Playback\"" "Rec Mode" {
      tunnel: w498 -> [_ _ w513]
      tunnel: [u32 2829099 ("Base Color") u32 11141120 ("Target Color") w502] -> w494
      frame "Stop", Default {
        # "Reset the color, extra updates don't cost much"
      }
      frame "Record" {
      }
      frame "Playback" {
        # "Playback"
        n322 = Quotient & Remainder(x=w513, y=u32 50 ("milliseconds to wait")) -> (x-y*floor(x/y)=w509:u32)  [unwired: 1 out]
        n323 = Divide(x=w509, y=u32 50 ("milliseconds to wait")) -> (x/y=w506:dbl)
        n324 = Multiply(x=6.283185307179586, y=w506) -> (x*y=w511:dbl)
        n325 = Sine(x=w511) -> (sin(x)=w510:dbl)
        n326 = Absolute Value(x=w510) -> (abs(x)=w503:dbl)
        n327 = call "Interpolate RGB Color.vi"("Proportion"=w503, "Target Color"=u32 30976, "Base Color"=u32 2829099) -> ("Result Color"=w502:u32)  [unwired: 8 in]
      }
    }
    n328 = property class="Pane"(reference=w495, "PaneColor"=w494) -> ()  [unwired: 1 in, 2 out]
  }
  n329 = local write "Dashboard Tab"(T2."Drive" ("Dashboard Tab")) -> ()
  n330 = property on="On/Off" class="Bool (strict)"("Visible"=w36) -> ()  [unwired: 2 in, 2 out]
  n331 = property on="Motor" class="Clust (strict)"("Visible"=w36) -> ()  [unwired: 2 in, 2 out]
  n332 = property on="Progress" class="Clust (strict)"("Visible"=w36) -> ()  [unwired: 2 in, 2 out]
  n333 = property on="Test Ring" class="Ring (strict)"("Visible"=w36) -> ()  [unwired: 2 in, 2 out]
  n334 = property on="Rev/Fwd" class="Clust (strict)"("Visible"=w36) -> ()  [unwired: 2 in, 2 out]
  n335 = while {
    tunnel: u16 1741 ("timeout ms (25000)") -> [w515]
    stop <- FALSE stop-if-true
    n336 = TCP Create Listener(10:w515) -> (0:w514:errorcluster, 3:w516:refnum<k5>)  [unwired: 4 in, 1 out]
    n337 = case shown="No Error" w514 {
      selector: w514 -> [w518 _]
      tunnel: w516 -> [w519 _]
      frame No Error {
        n338 = while {
          tunnel: w519 -> [w522]
          tunnel: w518 -> [w521]
          stop <- FALSE stop-if-true
          n339 = TCP Wait On Listener(8:w521, 11:w522) -> (0:w523:errorcluster, 4:w524:refnum<k5>)  [unwired: 2 in, 3 out]
          n340 = local write "TCP"(w524) -> ()
          n341 = case shown="No Error" w523 {
            frame No Error {
            }
            frame Error {
              n342 = Wait (ms)(milliseconds to wait=u32 1000) -> ()  [unwired: 1 out]
            }
          }
        }
      }
      frame Error {
        n343 = Wait (ms)(milliseconds to wait=u32 1000) -> ()  [unwired: 1 out]
      }
    }
  }
  n344 = local write "Command Selection"(u16 0 ("milliseconds to wait")) -> ()
  n345 = local write "Command Params"(string[][] [] ("Command Params")) -> ()
  n346 = global write "WPI_DashboardLogging Global.vi" "Recording"(w59) -> ()
  n347 = local write "Rec Mode"(w59) -> ()
  n348 = call <vilib>:"NT Write String.vi"("String"="Select Auto", "Name"="Auto Selector") -> ()  [unwired: 9 in, 1 out]
